vi "Apply.vi"(8 "Error In":errorcluster, 11 "Fetch Display CFG in":refnum<class "Fetch Display CFG.lvclass">) -> (0 "Error Out":errorcluster, 3 "Fetch Display CFG out":refnum<class "Fetch Display CFG.lvclass">)   [LabVIEW 2023, in "Fetch Display CFG.lvclass"]
uses:
  Fetch Display CFG.lvclass
  D:/git/LeCroy-HDO4000A-LabVIEW/Configurations/HDO4000A Base CFG/HDO4000A Base CFG.lvclass
  Fetch Display CFG.lvclass/Fetch Display CFG.ctl
  HDO4000A Base CFG/HDO4000A Base CFG.lvclass
  D:/git/HAL/Scope VISA/Configuration/Scope VISA CFG.lvclass
  D:/git/HAL/Configuration Base/Configuration Base.lvclass
  D:/git/HAL/Interfaces/IConfigure/IConfigure.lvclass
  D:/git/HAL/Interfaces/IConfigure Scope/IConfigure Scope.lvclass
  D:/git/LeCroy-HDO4000A-LabVIEW/Configurations/Fetch Display CFG/Fetch Display CFG.lvclass
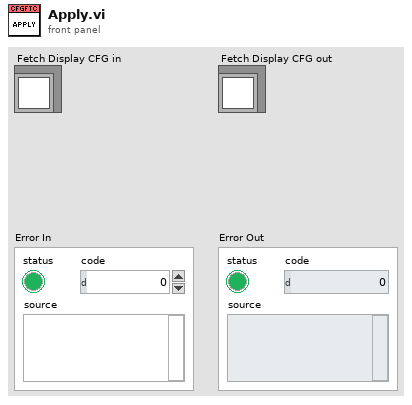
[diagram p1: front panel]
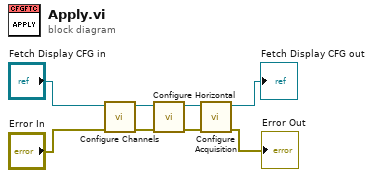
[diagram p0: block diagram]
diagram:
  n1 = call "Configure Channels.vi"("error in"="Error In", "HDO4000A Base CFG in"="Fetch Display CFG in") -> ("error out"=w7:errorcluster, "HDO4000A Base CFG out"=w5:refnum<class "Fetch Display CFG.lvclass">)  [unwired: 8 in]
  n2 = call "Configure Horizontal.vi"("error in"=w7, "HDO4000A Base CFG in"=w5) -> ("error out"=w3:errorcluster, "HDO4000A Base CFG out"=w4:refnum<class "Fetch Display CFG.lvclass">)  [unwired: 8 in]
  n3 = call-dynamic "Configure Acquisition.vi"("error in"=w3, "HDO4000A Base CFG in"=w4) -> ("error out"=→"Error Out":errorcluster, "HDO4000A Base CFG out"=→"Fetch Display CFG out":refnum<class "Fetch Display CFG.lvclass">)  [unwired: 8 in]
